vi "GetBusData.vi"(8 "Error In":errorcluster[](array[cluster]), 10 "arg":string, 11 "Bus in":refnum<class "Bus.lvclass">) -> (0 "Error Out":errorcluster[](array[cluster]), 2 "XmlData":string, 3 "Bus out":refnum<class "Bus.lvclass">)   [LabVIEW 2014, in "Bus_class.lvlib" / "Bus.lvclass"]
uses:
  Bus.lvclass
  Bus.lvclass/Bus.ctl
  Modules/EventModule/PublicAPI/Arguments/Requests/dblEvtParams.ctl
  Modules/EventPlugins/EventPluginBaseClass/TypeDefs/clEvtConfig.ctl
  Modules/EventPlugins/EventPluginBaseClass/TypeDefs/clEvtReportArray.ctl
  Modules/EventPlugins/EventPluginBaseClass/TypeDefs/clEvtReport.ctl
  Modules/EventPlugins/EventPluginBaseClass/TypeDefs/dblEvtSignalArray.ctl
  Modules/EventModule/PublicAPI/Arguments/Broadcasts/clErrorRpt.ctl
  Modules/PmuImpairPlugins/PmuImpairPluginBase_class/TypeDefs/clImpairConfig.ctl
  Modules/PmuImpairModule/PublicAPI/Arguments/Broadcasts/clErrorRpt.ctl
  Modules/NetworkImpairmentModule/PublicAPI/Arguments/Broadcasts/dblPktLoss.ctl
  Modules/NetworkImpairmentModule/PublicAPI/Arguments/Broadcasts/dblNetworkTime.ctl
  Modules/NetworkImpairmentModule/PublicAPI/Arguments/Broadcasts/clErrorRpt.ctl
  Modules/FlagImpairModule/PublicAPI/Arguments/Broadcasts/ui32FlagImpairmentArray.ctl
  <vilib>/Utility/error.llb/Error Cluster From Error Code.vi
  <vilib>/ErrorRing/Error Ring.xnode
  TestAutomation/LTA/LTA.lvlib
  <userlib>/NIST/NISTErrorLib/NISTErrorLib.lvlib
  Modules/EventModule/EventModule.lvlib
  Modules/EventPlugins/EventPluginBaseClass/EventPluginBaseClass.lvclass
  Modules/PmuImpairModule/PmuImpairModule.lvlib
  Modules/PmuImpairPlugins/PmuImpairPluginBase_class/PmuImpairPluginBase.lvclass
  Modules/NetworkImpairmentModule/NetworkImpairmentModule.lvlib
  Modules/FlagImpairModule/FlagImpairModule.lvlib
  Framework.lvlib
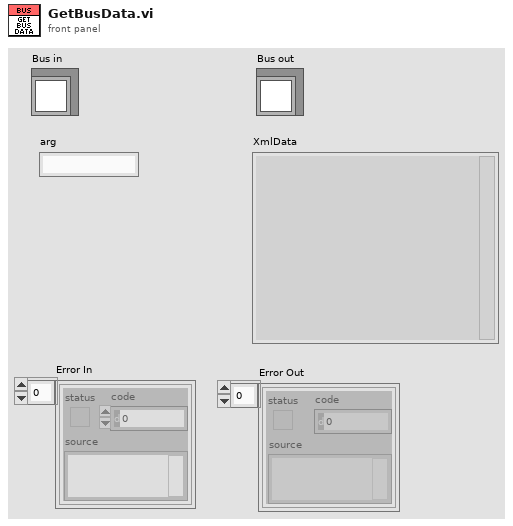
[diagram p1: front panel]
types:
  T1 = typedef "EventPlugins.lvlib/EventPluginBaseClass.lvclass/clEvtConfig.ctl" = cluster{"T0(UTC)":dbl, "F0":dbl, "Fs":i32, "FSamp":u32, "bPosSeq":bool}
  T2 = typedef "EventPlugins.lvlib/EventPluginBaseClass.lvclass/clEvtReportArray.ctl" = T3[]
  T3 = typedef "EventPlugins.lvlib/EventPluginBaseClass.lvclass/clEvtReport.ctl" = cluster{"Timestamp":dbl, "Synx":cdb[], "Freq":dbl, "ROCOF":dbl, "ID":i16}
  T4 = typedef "EventPlugins.lvlib/EventPluginBaseClass.lvclass/dblEvtSignalArray.ctl" = dbl[][]
  T5 = typedef "EventModule.lvlib/clErrorRpt.ctl" = cluster{"error":errorcluster, "AdditionalInfo":string}
  T6 = typedef "PmuImpairPlugins.lvlib/PmuImpairPluginBase.lvclass/clImpairConfig.ctl" = cluster{"FilterType":string, "bPosSeq":bool}
  T7 = typedef "PmuImpairModule.lvlib/clErrorRpt.ctl" = cluster{"error":errorcluster, "AdditionalInfo":string}
  T8 = typedef "EventModule.lvlib/dblEvtParams.ctl" = dbl[][]
  T9 = typedef "NetworkImpairmentModule.lvlib/clErrorRpt.ctl" = cluster{"error":errorcluster, "AdditionalInfo":string}
  T10 = typedef "EventModule.lvlib/clBroadcastEvents.ctl" = cluster{"DidInit":refnum<user-event>, "StatusUpdate":refnum<user-event>, "ErrorReport":refnum<user-event>, "DidStop":refnum<user-event>, "ReadEvtConfig":refnum<user-event>, "ReadTimeArray":refnum<user-event>, "ReadEvtParams":refnum<user-event>, "GetEvtReportArray":refnum<user-event>, "ReadPathToPlugin":refnum<user-event>, "GetEvtSignal":refnum<user-event>, "ReadBusNumber":refnum<user-event>}
  T11 = typedef "PmuImpairModule.lvlib/clBroadcastEvents.ctl" = cluster{"DidInit":refnum<user-event>, "StatusUpdate":refnum<user-event>, "ErrorReport":refnum<user-event>, "DidStop":refnum<user-event>, "ImpairConfig":refnum<user-event>, "ImpairParams":refnum<user-event>, "ImpairReports":refnum<user-event>, "PathToPlugin":refnum<user-event>, "BusNumber":refnum<user-event>}
  T12 = typedef "NetworkImpairmentModule.lvlib/clBroadcastEvents.ctl" = cluster{"DidInit":refnum<user-event>, "StatusUpdate":refnum<user-event>, "ErrorReport":refnum<user-event>, "DidStop":refnum<user-event>, "ReadNetImpParams":refnum<user-event>, "ReadLossThreshold":refnum<user-event>, "GetNetworkTime":refnum<user-event>, "GetPktLoss":refnum<user-event>, "ReadPathToPlugin":refnum<user-event>}
  T13 = typedef "NetworkImpairmentModule.lvlib/dblPktLoss.ctl" = dbl[]
  T14 = typedef "NetworkImpairmentModule.lvlib/dblNetworkTime.ctl" = dbl[]
  T15 = typedef "FlagImpairModule.lvlib/clBroadcastEvents.ctl" = cluster{"DidInit":refnum<user-event>, "StatusUpdate":refnum<user-event>, "ErrorReport":refnum<user-event>, "DidStop":refnum<user-event>, "ReadFlagImpairConfig":refnum<user-event>, "ReadPluginINIFilePath":refnum<user-event>, "ReadFlagImpairParams":refnum<user-event>, "ReadTimeArray":refnum<user-event>, "GetFlagImpairment":refnum<user-event>}
  T16 = typedef "FlagImpairModule.lvlib/ui32FlagImpairmentArray.ctl" = u32[]
  T17 = typedef "Framework.lvlib/clFrontPanelControlRefs.ctl" = cluster{"TestFilePathRef":refnum<vi>, "BusNumberRef":refnum<vi>, "NumberOfBusesRef":refnum<vi>, "EvtTypeRef":refnum<vi>, "EvtParamsRef":refnum<vi>, "EvtConfigRef":refnum<vi>, "StartTimeRef":refnum<vi>, "EndTimeRef":refnum<vi>, "PmuImpairTypeRef":refnum<vi>, "PmuImpairParamsRef":refnum<vi>, "NetImpairParamsRef":refnum<vi>, "FlagImpairTypeRef":refnum<vi>, "FlagImpairParamsRef":refnum<vi>, "NetImpairTypeRef":refnum<vi>, "OutputFileType":refnum<vi>, "PmuImpairConfigRef":refnum<vi>, "AppTypeRef":refnum<vi>, "ScriptPathRef":refnum<vi>, "ShowPanels?":refnum<vi>}
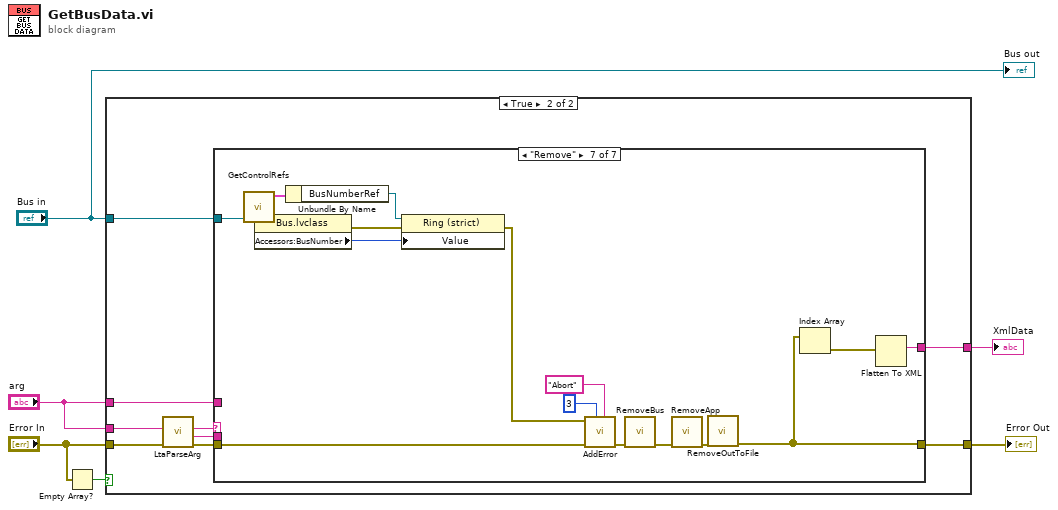
[diagram p0: block diagram]
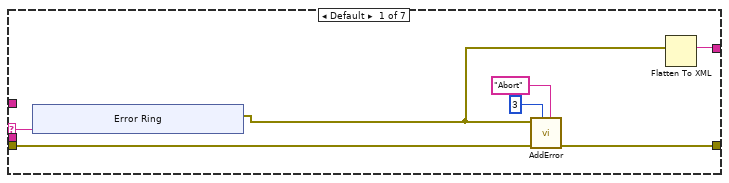
[diagram p3: hidden frame]
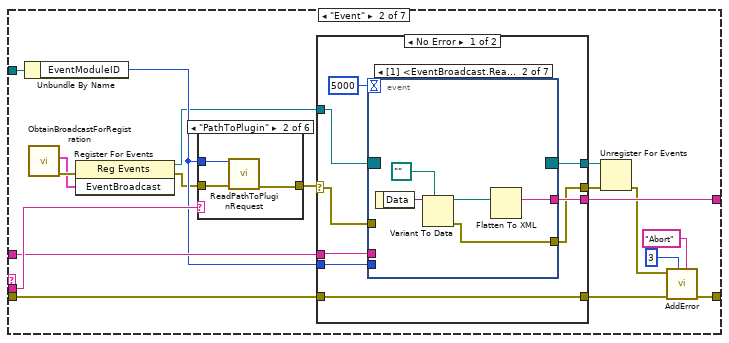
[diagram p4: hidden frame]
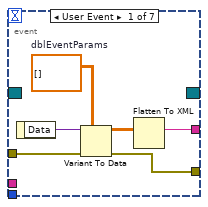
[diagram p5: hidden frame]
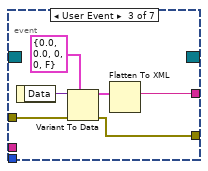
[diagram p6: hidden frame]
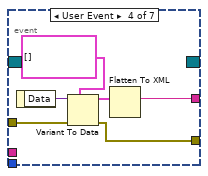
[diagram p7: hidden frame]
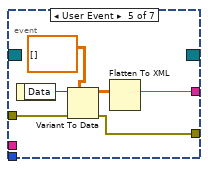
[diagram p8: hidden frame]
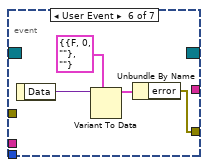
[diagram p9: hidden frame]
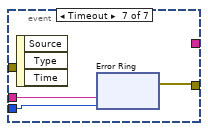
[diagram p10: hidden frame]
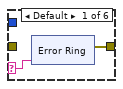
[diagram p12: hidden frame]
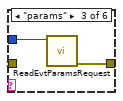
[diagram p13: hidden frame]
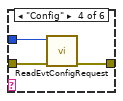
[diagram p14: hidden frame]
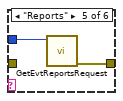
[diagram p15: hidden frame]
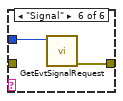
[diagram p16: hidden frame]
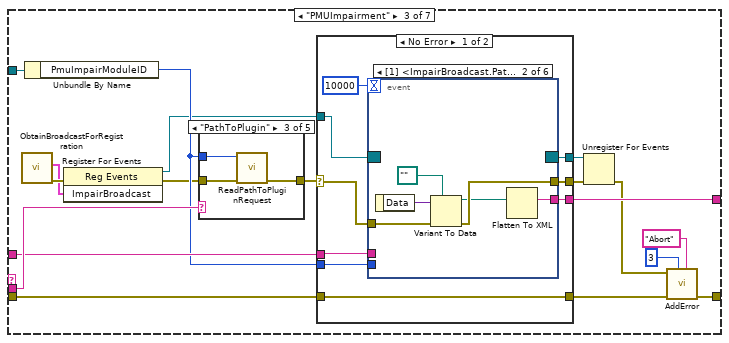
[diagram p17: hidden frame]
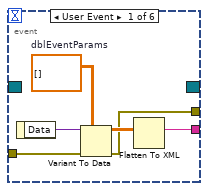
[diagram p18: hidden frame]
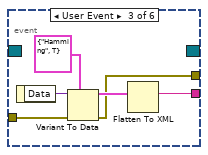
[diagram p19: hidden frame]
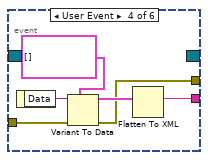
[diagram p20: hidden frame]
diagram:
  n1 = Empty Array?(array="Error In") -> (empty?=w6:bool)
  n2 = case shown="True" w6 {
    tunnel: "Bus in" -> [_ w10]
    tunnel: "Error In" -> [w7 w16]
    tunnel: [w7 w12] -> w4
    tunnel: "arg" -> [_ w15]
    tunnel: "arg" -> [_ w9]
    tunnel: [_ w8] -> w2
    frame False {
    }
    frame True {
      n3 = call "LtaParseArg.vi"("Error In"=w16, "Arg In"=w15) -> ("Error Out"=w13:errorcluster[], "ArgRemaining"=w11:string, "Arg 1"=w14:string)  [unwired: 6 in, 1 out]
      n4 = case shown="\"Remove\"" w14 {
        selector: w14 -> [w23 _ _ _ _ _ _]
        tunnel: w13 -> [w22 w45 w140 w230 w317 w387 w394]
        tunnel: [w21 w44 w139 w229 w316 w386 w390] -> w12
        tunnel: w11 -> [_ w47 w142 w232 w319 _ _]
        tunnel: w10 -> [_ w48 w143 w233 w320 _ w393]
        tunnel: w9 -> [_ w40 w135 w225 w312 _ _]
        tunnel: [w18 w39 w134 w224 w311 w389 w392] -> w8
        frame Default {
          n5 = xnode "Error Ring"("parameter 0"=w23) -> ("error out"=w17:errorcluster)
          n6 = call <userlib>:"AddError.vi"("Severity"="Abort", "Priority"=u8 3, "ErrorArray"=w22, "error in (no error)"=w17) -> ("ErrorArray"=w21:errorcluster[])  [unwired: 6 in, 1 out]
          n7 = Flatten To XML(anything=w17) -> (xml string=w18:string)
        }
        frame "Event" {
          n8 = Unbundle By Name(w48) -> ("EventModuleID"=w38:i32)
          n9 = call "ObtainBroadcastForRegistration.vi"() -> ("error out"=w37:errorcluster, "EventBroadcast"=w36:T10)  [unwired: 10 in]
          n10 = register-events(error in=w37, w36) -> (reference out=w31:refnum<event-registration>, error out=w35:errorcluster)  [unwired: 1 in]
          n11 = case shown="\"PathToPlugin\"" w47 {
            selector: w47 -> [w105 _ _ _ _ _]
            tunnel: [w106 w115 w118 w121 w123 w125] -> w46
            tunnel: w38 -> [_ w114 w117 w120 w122 w124]
            tunnel: w35 -> [_ w116 _ w119 _ _]
            frame Default {
              n12 = xnode "Error Ring"("parameter 0"=w105) -> ("error out"=w106:errorcluster)
            }
            frame "PathToPlugin" {
              n13 = call "ReadPathToPluginRequest.vi"("error in (no error)"=w116, "ModuleID"=w114) -> ("error out"=w115:errorcluster)  [unwired: 9 in]
            }
            frame "params" {
              n14 = call "ReadEvtParamsRequest.vi"("ModuleID"=w117) -> ("error out"=w118:errorcluster)  [unwired: 10 in]
            }
            frame "Config" {
              n15 = call "ReadEvtConfigRequest.vi"("error in (no error)"=w119, "ModuleID"=w120) -> ("error out"=w121:errorcluster)  [unwired: 9 in]
            }
            frame "Reports" {
              n16 = call "GetEvtReportsRequest.vi"("ModuleID"=w122) -> ("error out"=w123:errorcluster)  [unwired: 10 in]
            }
            frame "Signal" {
              n17 = call "GetEvtSignalRequest.vi"("ModuleID"=w124) -> ("error out"=w125:errorcluster)  [unwired: 10 in]
            }
          }
          n18 = case shown="No Error" w46 {
            selector: w46 -> [w50 w102]
            tunnel: w45 -> [w54 w104]
            tunnel: [w54 w104] -> w43
            tunnel: w40 -> [w57 _]
            tunnel: [w55 _] -> w39
            tunnel: w38 -> [w53 _]
            tunnel: [w52 w103] -> w34
            tunnel: [w51 w102] -> w33
            tunnel: w31 -> [w49 w103]
            frame No Error {
              n19 = event shown="[1] <EventBroadcast.ReadPathToPlugin>: User Event" {
                selector: w49 -> [_ _ _ _ _ _ _]
                dyn-events: [_ _ _ _ _ _ _] -> w52
                timeout: 5000 -> [_ _ _ _ _ _ _]
                tunnel: w50 -> [w62 _ w74 w80 w86 _ _]
                tunnel: [w61 w65 w70 w77 w83 w87 w93] -> w51
                tunnel: w57 -> [_ _ _ _ _ _ w92]
                tunnel: [w58 w66 w69 w76 w82 _ _] -> w55
                tunnel: w53 -> [_ _ _ _ _ _ w91]
                event User Event {
                  w60 = T8 []  # dblEventParams
                  n20 = event-data() -> ("Data"=w63:variant)  [unwired: 1 in]
                  n21 = Variant To Data(error in=w62, type=w60, Variant=w63) -> (data=w59:T8, error out=w61:errorcluster)
                  n22 = Flatten To XML(anything=w59) -> (xml string=w58:string)
                }
                event User Event {
                  n23 = event-data() -> ("Data"=w68:variant)  [unwired: 1 in]
                  n24 = Variant To Data(type=path "", Variant=w68) -> (data=w64:path, error out=w65:errorcluster)  [unwired: 1 in]
                  n25 = Flatten To XML(anything=w64) -> (xml string=w66:string)
                }
                event User Event {
                  n26 = event-data() -> ("Data"=w73:variant)  [unwired: 1 in]
                  n27 = Variant To Data(error in=w74, type=T1 {"T0(UTC)"=0.0, "F0"=0.0, "Fs"=0, "FSamp"=0, "bPosSeq"=FALSE} ("clEvtConfig"), Variant=w73) -> (data=w71:T1, error out=w70:errorcluster)
                  n28 = Flatten To XML(anything=w71) -> (xml string=w69:string)
                }
                event User Event {
                  n29 = event-data() -> ("Data"=w79:variant)  [unwired: 1 in]
                  n30 = Variant To Data(error in=w80, type=T2 [] ("clEvtReportArray"), Variant=w79) -> (data=w78:T2, error out=w77:errorcluster)
                  n31 = Flatten To XML(anything=w78) -> (xml string=w76:string)
                }
                event User Event {
                  n32 = event-data() -> ("Data"=w85:variant)  [unwired: 1 in]
                  n33 = Variant To Data(error in=w86, type=T4 [] ("dblEventSignalArray"), Variant=w85) -> (data=w84:T4, error out=w83:errorcluster)
                  n34 = Flatten To XML(anything=w84) -> (xml string=w82:string)
                }
                event User Event {
                  n35 = event-data() -> ("Data"=w88:variant)  [unwired: 1 in]
                  n36 = Variant To Data(type=T5 {"error"={"status"=FALSE, "code"=0, "source"=""}, "AdditionalInfo"=""} ("Cluster"), Variant=w88) -> (data=w89:T5)  [unwired: 1 in, 1 out]
                  n37 = Unbundle By Name(w89) -> ("error"=w87:errorcluster)
                }
                event Timeout {
                  n38 = event-data() -> ()  [unwired: 1 in, 3 out]
                  n39 = xnode "Error Ring"("parameter 0"=w92, "parameter 1"=w91) -> ("error out"=w93:errorcluster)
                }
              }
            }
            frame Error {
            }
          }
          n40 = Unregister For Events(event registration refnum=w34, error in=w33) -> (error out=w32:errorcluster)
          n41 = call <userlib>:"AddError.vi"("Severity"="Abort", "Priority"=u8 3, "ErrorArray"=w43, "error in (no error)"=w32) -> ("ErrorArray"=w44:errorcluster[])  [unwired: 6 in, 1 out]
        }
        frame "PMUImpairment" {
          n42 = call "ObtainBroadcastForRegistration.vi"() -> ("error out"=w131:errorcluster, "ImpairBroadcast"=w126:T11)  [unwired: 10 in]
          n43 = Unbundle By Name(w143) -> ("PmuImpairModuleID"=w133:i32)
          n44 = register-events(error in=w131, w126) -> (reference out=w127:refnum<event-registration>, error out=w132:errorcluster)  [unwired: 1 in]
          n45 = case shown="\"PathToPlugin\"" w142 {
            selector: w142 -> [w195 _ _ _ _]
            tunnel: [w196 w206 w209 w212 w215] -> w141
            tunnel: w133 -> [_ w205 w208 w211 w214]
            tunnel: w132 -> [_ w204 w207 w210 w213]
            frame Default {
              n46 = xnode "Error Ring"("parameter 0"=w195) -> ("error out"=w196:errorcluster)
            }
            frame "params" {
              n47 = call "ReadImpairParamsRequest.vi"("error in (no error)"=w204, "ModuleID"=w205) -> ("error out"=w206:errorcluster)  [unwired: 9 in]
            }
            frame "PathToPlugin" {
              n48 = call "ReadPathToPluginRequest.vi"("error in (no error)"=w207, "ModuleID"=w208) -> ("error out"=w209:errorcluster)  [unwired: 9 in]
            }
            frame "Config" {
              n49 = call "ReadImpairConfigRequest.vi"("error in (no error)"=w210, "ModuleID"=w211) -> ("error out"=w212:errorcluster)  [unwired: 9 in]
            }
            frame "Reports" {
              n50 = call "GetImpairReportsRequest.vi"("error in (no error)"=w213, "ModuleID"=w214) -> ("error out"=w215:errorcluster)  [unwired: 9 in]
            }
          }
          n51 = case shown="No Error" w141 {
            selector: w141 -> [w147 w193]
            tunnel: w140 -> [w149 w194]
            tunnel: [w149 w194] -> w138
            tunnel: w135 -> [w152 _]
            tunnel: [w150 _] -> w134
            tunnel: w133 -> [w148 _]
            tunnel: [w145 w193] -> w130
            tunnel: [w146 w192] -> w128
            tunnel: w127 -> [w144 w192]
            frame No Error {
              n52 = event shown="[1] <ImpairBroadcast.PathToPlugin>: User Event" {
                selector: w144 -> [_ _ _ _ _ _]
                dyn-events: [_ _ _ _ _ _] -> w146
                timeout: 10000 -> [_ _ _ _ _ _]
                tunnel: w147 -> [w157 w161 w170 w176 _ _]
                tunnel: w152 -> [_ _ _ _ _ w183]
                tunnel: [w154 w162 w166 w173 _ _] -> w150
                tunnel: w148 -> [_ _ _ _ _ w182]
                tunnel: [w153 w160 w165 w171 w177 w181] -> w145
                event User Event {
                  w156 = T8 []  # dblEventParams
                  n53 = event-data() -> ("Data"=w158:variant)  [unwired: 1 in]
                  n54 = Variant To Data(error in=w157, type=w156, Variant=w158) -> (data=w155:T8, error out=w153:errorcluster)
                  n55 = Flatten To XML(anything=w155) -> (xml string=w154:string)
                }
                event User Event {
                  n56 = event-data() -> ("Data"=w164:variant)  [unwired: 1 in]
                  n57 = Variant To Data(error in=w161, type=path "", Variant=w164) -> (data=w159:path, error out=w160:errorcluster)
                  n58 = Flatten To XML(anything=w159) -> (xml string=w162:string)
                }
                event User Event {
                  n59 = event-data() -> ("Data"=w169:variant)  [unwired: 1 in]
                  n60 = Variant To Data(error in=w170, type=T6 {"FilterType"="Hamming", "bPosSeq"=TRUE} ("clImpairConfig"), Variant=w169) -> (data=w167:T6, error out=w165:errorcluster)
                  n61 = Flatten To XML(anything=w167) -> (xml string=w166:string)
                }
                event User Event {
                  n62 = event-data() -> ("Data"=w175:variant)  [unwired: 1 in]
                  n63 = Variant To Data(error in=w176, type=T2 [] ("clEvtReportArray"), Variant=w175) -> (data=w174:T2, error out=w171:errorcluster)
                  n64 = Flatten To XML(anything=w174) -> (xml string=w173:string)
                }
                event User Event {
                  n65 = event-data() -> ("Data"=w178:variant)  [unwired: 1 in]
                  n66 = Variant To Data(type=T7 {"error"={"status"=FALSE, "code"=0, "source"=""}, "AdditionalInfo"=""} ("Cluster"), Variant=w178) -> (data=w179:T7)  [unwired: 1 in, 1 out]
                  n67 = Unbundle By Name(w179) -> ("error"=w177:errorcluster)
                }
                event Timeout {
                  n68 = event-data() -> ()  [unwired: 1 in, 3 out]
                  n69 = xnode "Error Ring"("parameter 0"=w183, "parameter 1"=w182) -> ("error out"=w181:errorcluster)
                }
              }
            }
            frame Error {
            }
          }
          n70 = Unregister For Events(event registration refnum=w128, error in=w130) -> (error out=w129:errorcluster)
          n71 = call <userlib>:"AddError.vi"("Severity"="Abort", "Priority"=u8 3, "ErrorArray"=w138, "error in (no error)"=w129) -> ("ErrorArray"=w139:errorcluster[])  [unwired: 6 in, 1 out]
        }
        frame "NetImpairment" {
          n72 = Unbundle By Name(w233) -> ("NetworkImpairModuleID"=w223:i32)
          n73 = call "ObtainBroadcastForRegistration.vi"() -> ("error out"=w219:errorcluster, "NetImpBroadcast"=w218:T12)  [unwired: 10 in]
          n74 = register-events(error in=w219, w218) -> (reference out=w217:refnum<event-registration>, error out=w220:errorcluster)  [unwired: 1 in]
          n75 = case shown="\"PathToPlugin\"" w232 {
            selector: w232 -> [w285 _ _ _ _]
            tunnel: [w286 w294 w297 w300 w302] -> w231
            tunnel: w223 -> [_ _ w296 w299 w301]
            tunnel: w220 -> [_ w295 _ w298 _]
            frame Default {
              n76 = xnode "Error Ring"("parameter 0"=w285) -> ("error out"=w286:errorcluster)
            }
            frame "PathToPlugin" {
              n77 = call "ReadPathToPluginRequest.vi"("error in (no error)"=w295) -> ("error out"=w294:errorcluster)  [unwired: 10 in]
            }
            frame "params" {
              n78 = call "ReadNetImpParamsRequest.vi"("ModuleID"=w296) -> ("error out"=w297:errorcluster)  [unwired: 10 in]
            }
            frame "PktLoss" {
              n79 = call "GetPktLossRequest.vi"("error in (no error)"=w298, "ModuleID"=w299) -> ("error out"=w300:errorcluster)  [unwired: 9 in]
            }
            frame "Reports" {
              n80 = call "GetNetTimeRequest.vi"("ModuleID"=w301) -> ("error out"=w302:errorcluster)  [unwired: 10 in]
            }
          }
          n81 = case shown="No Error" w231 {
            selector: w231 -> [w234 w282]
            tunnel: w230 -> [w239 w284]
            tunnel: [w239 w284] -> w228
            tunnel: w225 -> [w242 _]
            tunnel: [w240 _] -> w224
            tunnel: w223 -> [w238 _]
            tunnel: [w237 w283] -> w222
            tunnel: [w236 w282] -> w221
            tunnel: w217 -> [w235 w283]
            frame No Error {
              n82 = event shown="[1] <NetImpBroadcast.ReadPathToPlugin>: User Event" {
                selector: w235 -> [_ _ _ _ _ _]
                dyn-events: [_ _ _ _ _ _] -> w237
                timeout: 5000 -> [_ _ _ _ _ _]
                tunnel: w234 -> [w243 w250 w260 w266 _ _]
                tunnel: [w247 w251 w257 w264 w267 w273] -> w236
                tunnel: w242 -> [_ _ _ _ _ w272]
                tunnel: [w244 w252 w256 w263 _ _] -> w240
                tunnel: w238 -> [_ _ _ _ _ w271]
                event User Event {
                  n83 = event-data() -> ("Data"=w248:variant)  [unwired: 1 in]
                  n84 = Variant To Data(error in=w243, type=T8 [] ("dblEventParams"), Variant=w248) -> (data=w245:T8, error out=w247:errorcluster)
                  n85 = Flatten To XML(anything=w245) -> (xml string=w244:string)
                }
                event User Event {
                  n86 = event-data() -> ("Data"=w254:variant)  [unwired: 1 in]
                  n87 = Variant To Data(error in=w250, type=path "", Variant=w254) -> (data=w249:path, error out=w251:errorcluster)
                  n88 = Flatten To XML(anything=w249) -> (xml string=w252:string)
                }
                event User Event {
                  w255 = T13 []  # dblPktLoss
                  n89 = event-data() -> ("Data"=w259:variant)  [unwired: 1 in]
                  n90 = Variant To Data(error in=w260, type=w255, Variant=w259) -> (data=w258:T13, error out=w257:errorcluster)
                  n91 = Flatten To XML(anything=w258) -> (xml string=w256:string)
                }
                event User Event {
                  w262 = T14 []  # dblNetworkTime
                  n92 = event-data() -> ("Data"=w261:variant)  [unwired: 1 in]
                  n93 = Variant To Data(error in=w266, type=w262, Variant=w261) -> (data=w265:T14, error out=w264:errorcluster)
                  n94 = Flatten To XML(anything=w265) -> (xml string=w263:string)
                }
                event User Event {
                  n95 = event-data() -> ("Data"=w268:variant)  [unwired: 1 in]
                  n96 = Variant To Data(type=T9 {"error"={"status"=FALSE, "code"=0, "source"=""}, "AdditionalInfo"=""} ("Cluster"), Variant=w268) -> (data=w269:T9)  [unwired: 1 in, 1 out]
                  n97 = Unbundle By Name(w269) -> ("error"=w267:errorcluster)
                }
                event Timeout {
                  n98 = event-data() -> ()  [unwired: 1 in, 3 out]
                  n99 = xnode "Error Ring"("parameter 0"=w272, "parameter 1"=w271) -> ("error out"=w273:errorcluster)
                }
              }
            }
            frame Error {
            }
          }
          n100 = Unregister For Events(event registration refnum=w222, error in=w221) -> (error out=w216:errorcluster)
          n101 = call <userlib>:"AddError.vi"("Severity"="Abort", "Priority"=u8 3, "ErrorArray"=w228, "error in (no error)"=w216) -> ("ErrorArray"=w229:errorcluster[])  [unwired: 6 in, 1 out]
        }
        frame "FlagImpairment" {
          n102 = Unbundle By Name(w320) -> ("FlagImpairModuleID"=w310:i32)
          n103 = call "ObtainBroadcastForRegistration.vi"() -> ("error out"=w304:errorcluster, "FlagImpairBroadcasts"=w303:T15)  [unwired: 10 in]
          n104 = register-events(error in=w304, w303) -> (reference out=w305:refnum<event-registration>, error out=w306:errorcluster)  [unwired: 1 in]
          n105 = case shown="\"PathToPlugin\"" w319 {
            selector: w319 -> [w366 _ _ _ _]
            tunnel: [w367 w376 w380 w382 w384] -> w318
            tunnel: w310 -> [_ w375 w379 w381 w383]
            tunnel: w306 -> [_ w377 w378 _ _]
            frame Default {
              n106 = xnode "Error Ring"("parameter 0"=w366) -> ("error out"=w367:errorcluster)
            }
            frame "PathToPlugin" {
              n107 = call "ReadPluginINIFilePathRequest.vi"("error in (no error)"=w377, "ModuleID"=w375) -> ("error out"=w376:errorcluster)  [unwired: 9 in]
            }
            frame "params" {
              n108 = call "ReadFlagImpairParamsRequest.vi"("error in (no error)"=w378, "ModuleID"=w379) -> ("error out"=w380:errorcluster)  [unwired: 9 in]
            }
            frame "FlagImpairArray" {
              n109 = call "GetFlagImpairmentArrayRequest.vi"("ModuleID"=w381) -> ("error out"=w382:errorcluster)  [unwired: 10 in]
            }
            frame "Reports" {
              n110 = call "GetNetTimeRequest.vi"("ModuleID"=w383) -> ("error out"=w384:errorcluster)  [unwired: 10 in]
            }
          }
          n111 = case shown="No Error" w318 {
            selector: w318 -> [w321 w364]
            tunnel: w317 -> [w326 w365]
            tunnel: [w326 w365] -> w315
            tunnel: w312 -> [w329 _]
            tunnel: [w327 _] -> w311
            tunnel: w310 -> [w325 _]
            tunnel: [w324 w363] -> w309
            tunnel: [w323 w364] -> w308
            tunnel: w305 -> [w322 w363]
            frame No Error {
              n112 = event shown="[1] <FlagImpairBroadcasts.ReadPluginINIFilePath>: User Event" {
                selector: w322 -> [_ _ _ _ _]
                dyn-events: [_ _ _ _ _] -> w324
                timeout: 5000 -> [_ _ _ _ _]
                tunnel: w321 -> [w334 w337 w347 _ _]
                tunnel: [w333 w338 w344 w348 w354] -> w323
                tunnel: w329 -> [_ _ _ _ w353]
                tunnel: [w330 w339 w343 _ _] -> w327
                tunnel: w325 -> [_ _ _ _ w352]
                event User Event {
                  n113 = event-data() -> ("Data"=w335:variant)  [unwired: 1 in]
                  n114 = Variant To Data(error in=w334, type=T8 [] ("dblEventParams"), Variant=w335) -> (data=w331:T8, error out=w333:errorcluster)
                  n115 = Flatten To XML(anything=w331) -> (xml string=w330:string)
                }
                event User Event {
                  n116 = event-data() -> ("Data"=w341:variant)  [unwired: 1 in]
                  n117 = Variant To Data(error in=w337, type=path "", Variant=w341) -> (data=w336:path, error out=w338:errorcluster)
                  n118 = Flatten To XML(anything=w336) -> (xml string=w339:string)
                }
                event User Event {
                  w342 = T16 []  # ui32FlagImpairmentArray
                  n119 = event-data() -> ("Data"=w346:variant)  [unwired: 1 in]
                  n120 = Variant To Data(error in=w347, type=w342, Variant=w346) -> (data=w345:T16, error out=w344:errorcluster)
                  n121 = Flatten To XML(anything=w345) -> (xml string=w343:string)
                }
                event User Event {
                  n122 = event-data() -> ("Data"=w349:variant)  [unwired: 1 in]
                  n123 = Variant To Data(type=T9 {"error"={"status"=FALSE, "code"=0, "source"=""}, "AdditionalInfo"=""} ("Cluster"), Variant=w349) -> (data=w350:T9)  [unwired: 1 in, 1 out]
                  n124 = Unbundle By Name(w350) -> ("error"=w348:errorcluster)
                }
                event Timeout {
                  n125 = event-data() -> ()  [unwired: 1 in, 3 out]
                  n126 = xnode "Error Ring"("parameter 0"=w353, "parameter 1"=w352) -> ("error out"=w354:errorcluster)
                }
              }
            }
            frame Error {
            }
          }
          n127 = Unregister For Events(event registration refnum=w309, error in=w308) -> (error out=w307:errorcluster)
          n128 = call <userlib>:"AddError.vi"("Severity"="Abort", "Priority"=u8 3, "ErrorArray"=w315, "error in (no error)"=w307) -> ("ErrorArray"=w316:errorcluster[])  [unwired: 6 in, 1 out]
        }
        frame "Add" {
          n129 = call "Enqueue.vi"("ErrorArray"=w387, "Msg"="UpdateBusFromFrontPanel") -> ("ErrorArray"=w386:errorcluster[])  [unwired: 9 in]
          n130 = Index Array(array=w386) -> (element=w388:errorcluster)  [unwired: 1 in]
          n131 = Flatten To XML(anything=w388) -> (xml string=w389:string)
        }
        frame "Remove" {
          n132 = call "GetControlRefs.vi"() -> ("clControlRefs Out"=w397:T17)  [unwired: 11 in]
          n133 = property class="Bus.lvclass"(reference=w393) -> (error out=w400:errorcluster, "Accessors:BusNumber"=w399:u8)  [unwired: 1 in, 1 out]
          n134 = Unbundle By Name(w397) -> ("BusNumberRef"=w398:refnum<vi>)
          n135 = property class="Ring (strict)"(reference=w398, error in=w400, "Value"=w399) -> (error out=w402:errorcluster)  [unwired: 1 out]
          n136 = call <userlib>:"AddError.vi"("Severity"="Abort", "Priority"=u8 3, "ErrorArray"=w394, "error in (no error)"=w402) -> ("ErrorArray"=w401:errorcluster[])  [unwired: 6 in, 1 out]
          n137 = call "RemoveBus.vi"("ErrorArray In"=w401) -> ("ErrorArray Out"=w395:errorcluster[])  [unwired: 10 in]
          n138 = call "RemoveApp.vi"("ErrorArray In"=w395) -> ("ErrorArray Out"=w396:errorcluster[])  [unwired: 10 in]
          n139 = call "RemoveOutToFile.vi"("ErrorArray In"=w396) -> ("ErrorArray Out"=w390:errorcluster[])  [unwired: 10 in]
          n140 = Index Array(array=w390) -> (element=w391:errorcluster)  [unwired: 1 in]
          n141 = Flatten To XML(anything=w391) -> (xml string=w392:string)
        }
      }
    }
  }
  "Error Out" <- w4
  "XmlData" <- w2
  "Bus out" <- "Bus in"
